vi "Reset Supply.vi"(8 "error in":errorcluster, 11 "36234A in":refnum<class "36234A.lvclass">) -> (0 "error out":errorcluster, 3 "36234A out":refnum<class "36234A.lvclass">)   [LabVIEW 2019, in "36234A.lvlib" / "36234A.lvclass"]
uses:
  Library/36234A.lvclass
  Library/36234A.lvclass/36234A.ctl
  builds/Instruments/PowerSupply.lvlibp/Library/PowerSupply.lvclass
  <instrlib>/Keysight E36000 Series/Keysight E36000 Series.lvlib
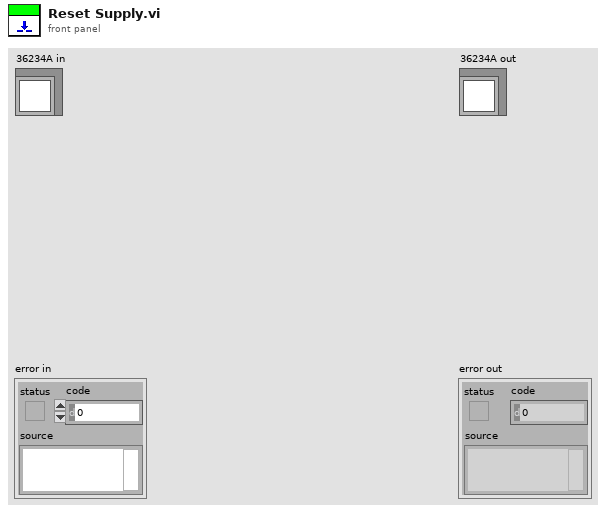
[diagram p1: front panel]
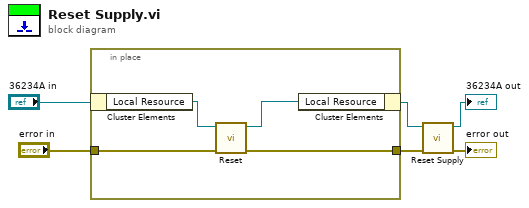
[diagram p0: block diagram]
diagram:
  n1 = in-place {
    in-place-border: "error in" -> [w10]
    in-place-border: [w7] -> w2
    n2 = in-place-cluster #1("36234A in") -> ("Local Resource"=w9:refnum<visa-resource-name>)
    n3 = call <instrlib>:"Reset.vi"("error in (no error)"=w10, "VISA resource name"=w9) -> ("error out"=w7:errorcluster, "VISA resource name out"=w8:refnum<visa-resource-name>)  [unwired: 8 in]
    n4 = in-place-cluster #1("Local Resource"=w8) -> (w1:refnum<class "36234A.lvclass">)
  }
  n5 = call-parent "Reset Supply.vi"("error in"=w2, "PowerSupply in"=w1) -> ("error out"=→"error out":errorcluster, "PowerSupply out"=→"36234A out":refnum<class "36234A.lvclass">)  [unwired: 8 in]
